vi "Get Mode.vi"(8 "error in (no error)":errorcluster, 11 "Inst.FP in":refnum<class "Inst.FP.lvclass">) -> (0 "error out":errorcluster, 2 "Mode":T1, 3 "Inst.FP out":refnum<class "Inst.FP.lvclass">)   [LabVIEW 2019, in "Inst.FP.lvclass"]
uses:
  Inst.FP.lvclass
  Typedefs/Inst.FP.Modes--Enum.ctl
  Typedefs/Inst.FP.Get Mode--Cluster.ctl
  d5aeea22-43ef-4aeb-99ea-2317f764c5f3.vi
  Typedefs/Inst.FP.Commands--Enum.ctl
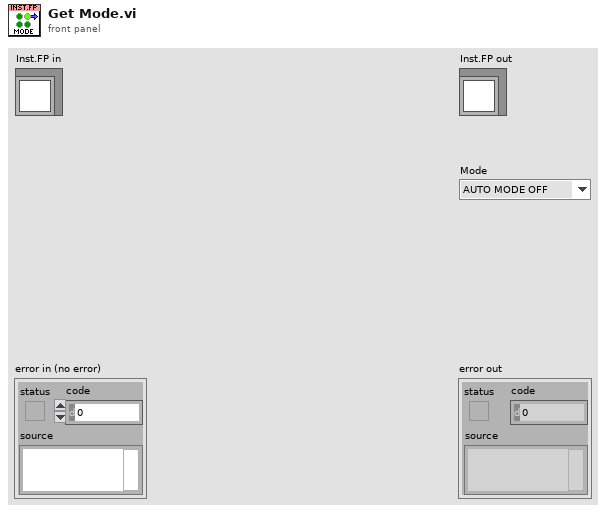
[diagram p1: front panel]
types:
  T1 = typedef "Inst.FP.lvclass/Inst.FP.Modes--Enum.ctl" = enum16{"AUTO MODE OFF", "START", "CONDENSING 3He", "CONDENSING 4He", "NORMAL CIRCULATION", "RECOVERY OF THE MIXTURE", "RECOVERY: BLOCKAGE or OVERPRESSURE"}
  T2 = typedef "Inst.FP.lvclass/Inst.FP.Commands--Enum.ctl" = enum16{"Get Mode", "Set Mode", "Push Button"}
  T3 = typedef "Inst.FP.lvclass/Inst.FP.Get Mode--Cluster.ctl" = cluster{"Mode":T1}
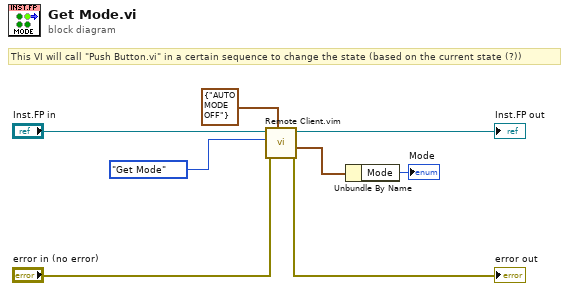
[diagram p0: block diagram]
diagram:
  # "This VI will call \"Push Button.vi\" in a certain sequence to change the state (based on the current state (?))"
  n1 = call "Remote Client.vim"("Data Out type"=T3 {"Mode"=enum."AUTO MODE OFF"} ("Get Mode"), "error in (no error)"="error in (no error)", "method"=Inst.FP.Commands--Enum."Get Mode" ("Commands"), "Instrument in"="Inst.FP in") -> ("error out"=→"error out":errorcluster, "Data out"=w2:T3, "Instrument out"=→"Inst.FP out":refnum<class "Inst.FP.lvclass">)  [unwired: 4 in, 1 out]
  n2 = Unbundle By Name(w2) -> ("Mode"=→"Mode":T1)
